vi "oa_History Pulse Processing.vi"(9 "pulse history in [s]":dbl[](array[numeric]) format="%.2f", 10 "pulse new history in  [s]":dbl[](array[numeric]) format="%.2f", 11 "pulse positions [s]":dbl[](array[numeric]) format="%.2f") -> (1 "pulse history out [s]":dbl[](array[numeric]) format="%.2f")   [LabVIEW 2017, in "SoundVib_TachProcess.lvlib"]
uses:
  <vilib>/addons/Sound and Vibration/Order Analysis/Tach Process/SoundVib_TachProcess.lvlib
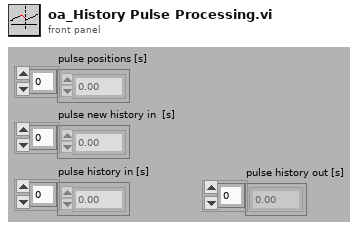
[diagram p1: front panel]
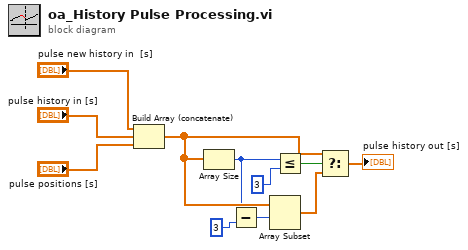
[diagram p0: block diagram]
diagram:
  n1 = Build Array (concatenate)("pulse new history in  [s]", "pulse history in [s]", "pulse positions [s]") -> (w3:dbl[])
  n2 = Array Size(array=w3) -> (size(s)=w2:i32)
  n3 = Subtract(x=w2, y=3) -> (x-y=w6:i32)
  n4 = Array Subset(array=w3, index=w6) -> (w5:dbl[])  [unwired: 1 in]
  n5 = Less Or Equal?(x=w2, y=3) -> (x <= y?=w4:bool)
  n6 = Select(t=w3, s=w4, f=w5) -> (s? t:f=→"pulse history out [s]":dbl[])
